vi "R30_1-RT.vi"() -> ()   [LabVIEW 2016]
uses:
  Controls/GP307 cluster.ctl
  Controls/Aperture states.ctl
  Controls/Faraday cup states.ctl
  Controls/Cryo Readback.ctl
  <vilib>/FPGAPlugInAG/cRIO-9067/niLvFpga_Open_cRIO-9067.vi
  <vilib>/rvi/interface/common/dynamic/niFpgaDynamicAddResources.vi
  <vilib>/Utility/error.llb/Error Cluster From Error Code.vi
  <vilib>/rvi/errors/niLvFpgaAdjustHostInterfaceError.vi
  <vilib>/rvi/interface/nirviOpenFPGA/nirviOpenFPGA.xnode
  PRIME Lab 2017a/Builds/cRIOs/R30-cRIO/FPGA/PRIMEControl2017_FPGA-R30_FPGA-R30_glZcTR5UBYc.lvbitx
  PRIME Lab 2017a/CONnie/PRIME Control 2017a/cRIO code/R30-1/R30_1-FPGA.vi
  <vilib>/rvi/interface/nirviReadWriteControl/nirviReadWriteControl.xnode
  <vilib>/NI_Real-Time Target Support.lvlib
  <vilib>/rvi/interface/Simulation/niFpgaSimulationCallBeginRW.vi
  NiFpgaLv.dll
panel:
  out "X+ Steerer V set":fxp<+/-,20,5>
  out "X- Steerer V set":fxp<+/-,20,5>
  out "Y+ Steerer V set":fxp<+/-,20,5>
  out "Y- Steerer V set":fxp<+/-,20,5>
  out "Cryo Readback":T1
  out "Time since re-purge":string
  out "2nd Stage Temp":string
  out "1st Stage Temp":string
  out "On-time":string
  out "Status":string
  in  "Tab Control":T2(tab)
  out "ESA I read":fxp<+/-,26,5>
  out "ESA V read":fxp<+/-,26,7>
  out "X- Steerer V read":fxp<+/-,26,7>
  out "Y+ Steerer I read":fxp<+/-,26,5>
  out "Y+ Steerer V read":fxp<+/-,26,7>
  out "Y- Steerer I read":fxp<+/-,26,5>
  out "Y- Steerer V read":fxp<+/-,26,7>
  out "X+ Steerer V read":fxp<+/-,26,7>
  out "X- Steerer I read":fxp<+/-,26,5>
  out "X+ Steerer I read":fxp<+/-,26,5>
  out "ESA Voltage set":fxp<+/-,20,5>
  out "Quad B I read":fxp<+/-,26,5>
  out "Quad A I read":fxp<+/-,26,5>
  out "Quad A set":fxp<+/-,20,5>
  out "Quad B set":fxp<+/-,20,5>
  out "Mag Steerer I-program":fxp<+/-,20,5>
  out "Mag Steerer V read":fxp<+/-,26,7>
  out "Mag Steerer I read":fxp<+/-,26,5>
  out "R30 Detector Ion gauge 1":u8[](array[numeric])
  out "R30 Detector Convectron  1":u8[](array[numeric])
  out "R30 ESA Ion gauge 1":u8[](array[numeric])
  out "Switch Image Convectron 1":u8[](array[numeric])
  out "Switch Image Ion Gauge 1":u8[](array[numeric])
  out "R30 ESA Convectron  1":u8[](array[numeric])
  out "Cryo 1st stage temp":u8[](array[numeric])
  out "Cryo On-time":u8[](array[numeric])
  out "Cryo status":u8[](array[numeric])
  out "Cryo 2nd stage temp":u8[](array[numeric])
  out "Time since repurge":u8[](array[numeric])
  out "ESA Vac cluster":T3
  out "Switch Image Vac Cluster":T3
  out "Detector Vac Cluster":T3
  out "Detector FC Status":T4
  out "Switch Image FC Status":T4
  out "Switch Image Aperture Status":T5
  out "Detector FC Position":cluster{"IN sensor":bool, "OUT sensor":bool}
  out "Detector Aperture Status":T5
  out "Switch Image FC Position":cluster{"IN sensor":bool, "OUT sensor":bool}
  out "Switch Image Aperture Position":cluster{"IN sensor":bool, "OUT sensor":bool}
  out "Detector Aperture Position":cluster{"IN sensor":bool, "OUT sensor":bool}
  out "Error Reporter":errorcluster
  out "HV control loop error":errorcluster
  out "HV readback loop error":errorcluster
  out "Actuator Sensor loop error":errorcluster
  out "Vac Cluster loop error":errorcluster
  out "Cryo loop error":errorcluster
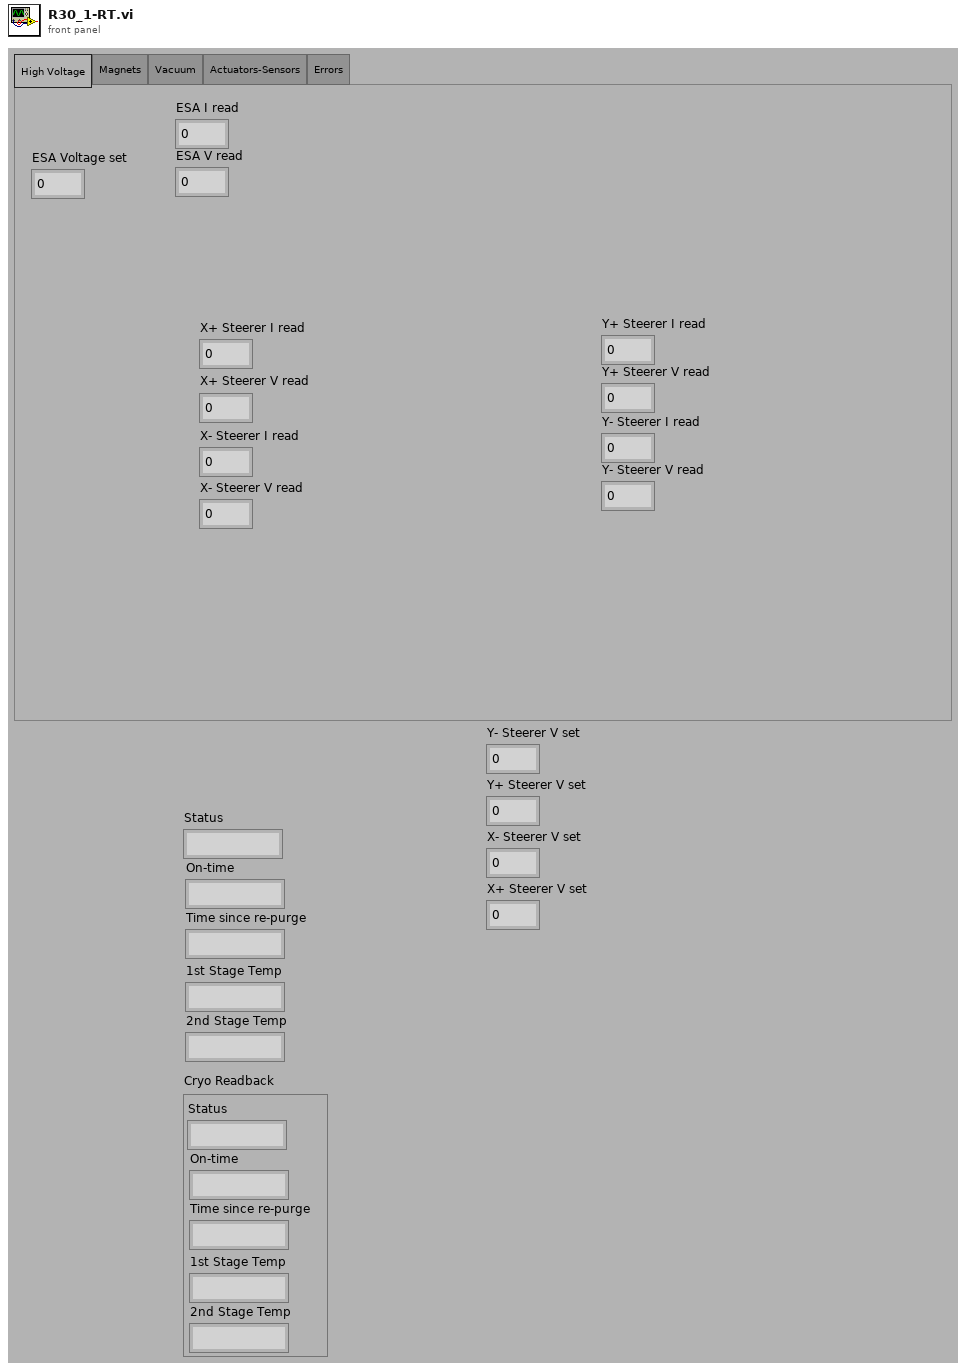
[diagram p1: front panel]
types:
  T1 = typedef "Cryo Readback.ctl" = cluster{"Status":string, "On-time":string, "1st Stage Temp":string, "2nd Stage Temp":string, "Time since re-purge":string}
  T2 = enum32{"High Voltage", "Magnets", "Vacuum", "Actuators-Sensors", "Errors"}
  T3 = typedef "GP307 cluster.ctl" = cluster{"Ion gauge 1":string, "Convectron  Gauge 1 ":string, "Ion Gauge 2":string, "Convectrom Gauge 2":string}
  T4 = typedef "Faraday cup states.ctl" = enum16{"FC status unclear", "FC in", "FC out"}
  T5 = typedef "Aperture states.ctl" = enum16{"Aperture status unclear", "Aperture in", "Aperture out"}
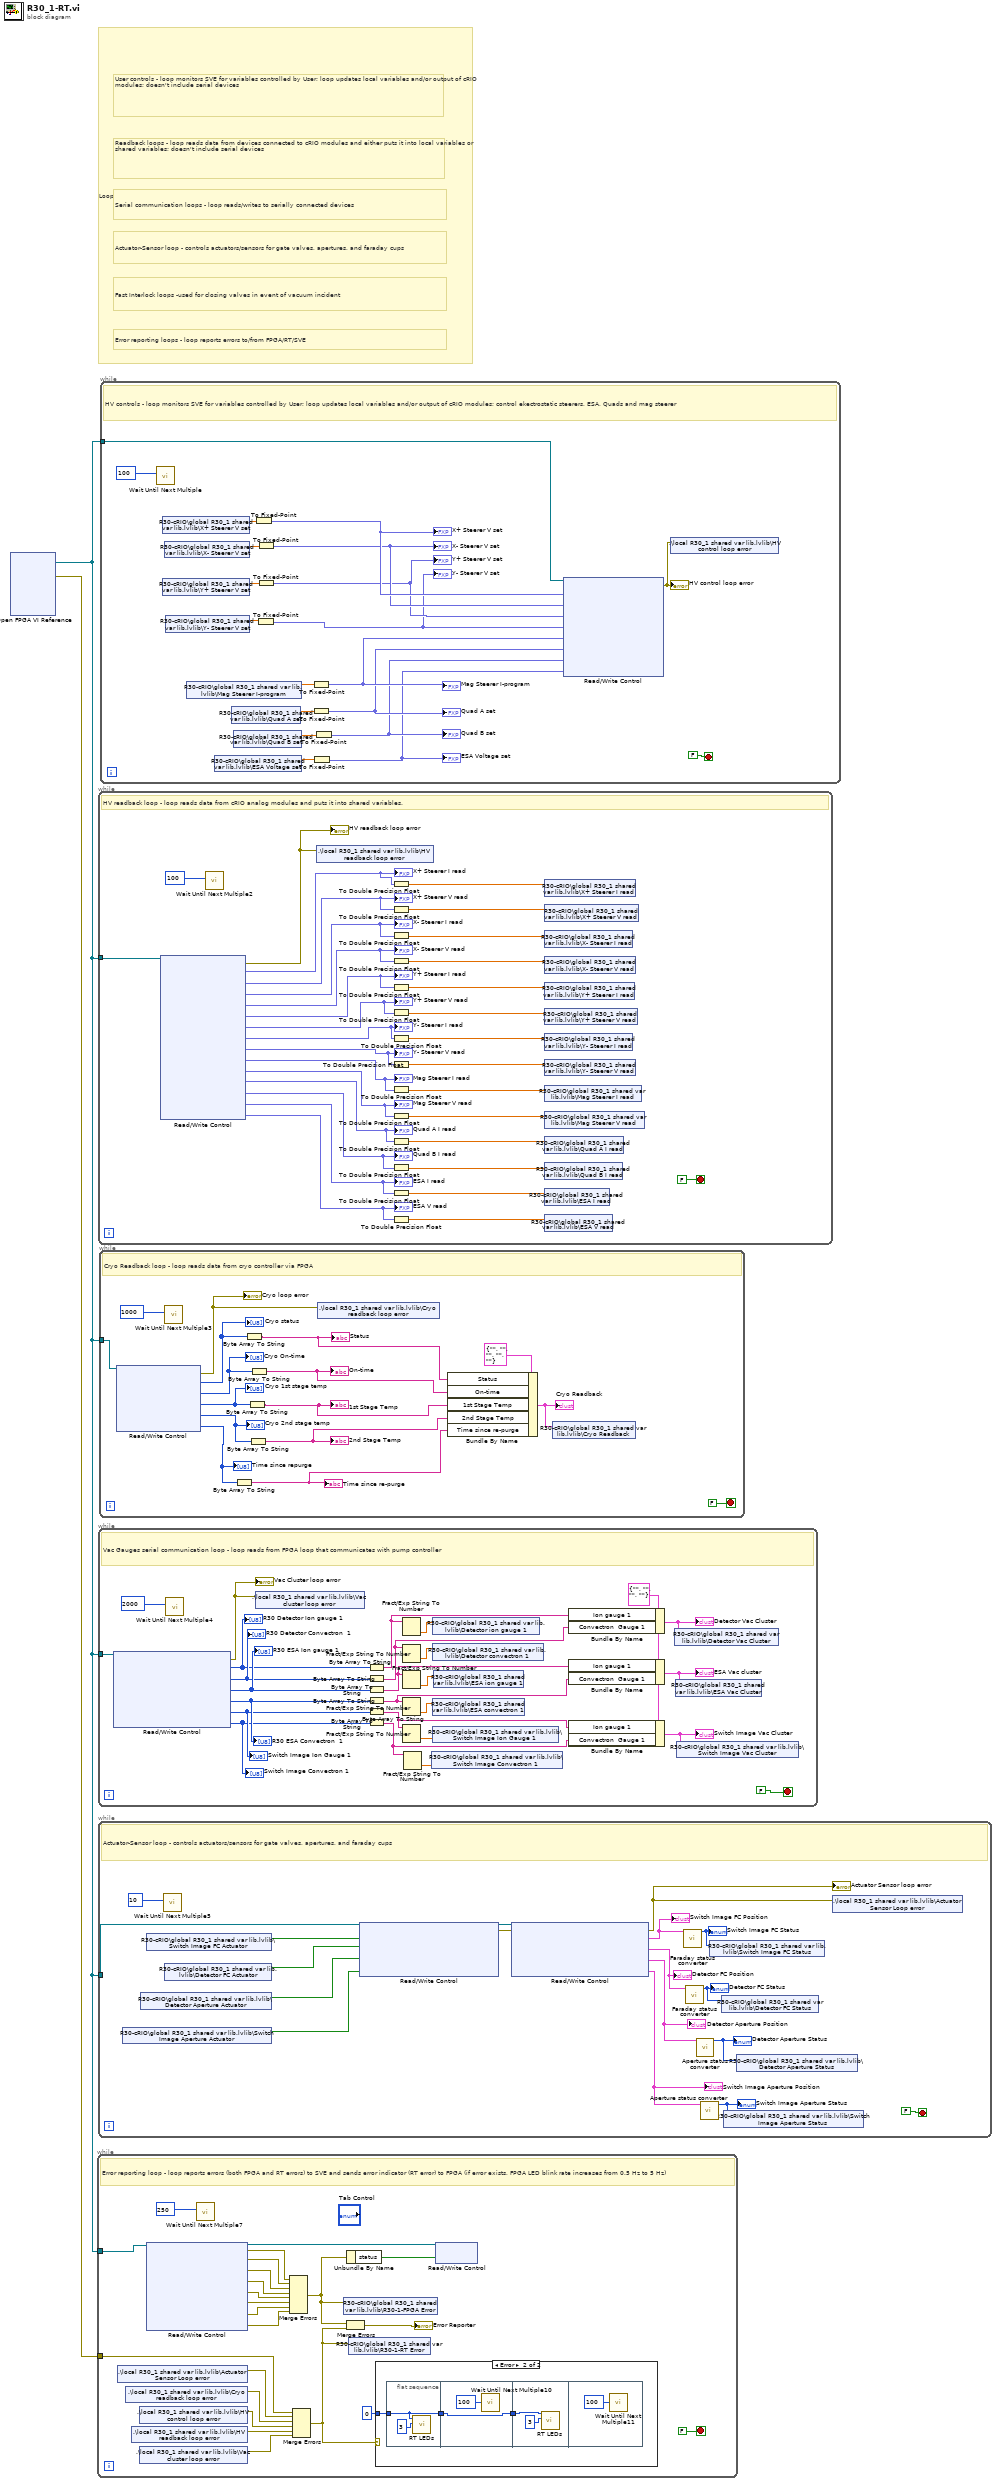
[diagram p0: block diagram]
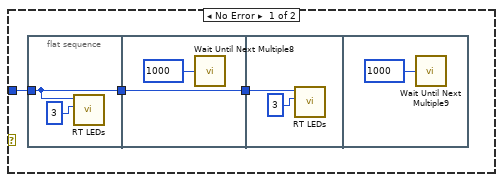
[diagram p2: hidden frame]
diagram:
  # "Actuator-Sensor loop - controls actuators/sensors for gate valves, apertures, and faraday cups"
  # "Fast Interlock loops -used for closing valves in event of vacuum incident"
  # "Error reporting loops - loop reports errors to/from FPGA/RT/SVE"
  # "Serial communication loops - loop reads/writes to serially connected devices"
  # "Readback loops - loop reads data from devices connected to cRIO modules and either puts it into local variables or shared variables; doesn't include serial devices"
  # "User controls - loop monitors SVE for variables controlled by User; loop updates local variables and/or output of cRIO modules; doesn't include serial devices"
  # "Loop legend - loops are color coded by responsibility"
  n1 = xnode "Open FPGA VI Reference"() -> ("FPGA VI Reference Out"=w1:refnum<k20>, "error out"=w2:errorcluster)  [unwired: 2 in]
  n2 = while {
    tunnel: w1 -> [w25]
    tunnel: w2 -> [w5]
    stop <- FALSE stop-if-true
    # "Error reporting loop - loop reports errors (both FPGA and RT errors) to SVE and sends error indicator (RT error) to FPGA (if error exists, FPGA LED blink rate increases from 0.5 Hz to 5 Hz)"
    n3 = shared-variable ".\\local R30_1 shared var lib.lvlib\\Actuator Sensor Loop error"() -> (w6:errorcluster)  [unwired: 1 in, 1 out]
    n4 = shared-variable ".\\local R30_1 shared var lib.lvlib\\Cryo readback loop error"() -> (w7:errorcluster)  [unwired: 1 in, 1 out]
    n5 = shared-variable ".\\local R30_1 shared var lib.lvlib\\HV readback loop error"() -> (w9:errorcluster)  [unwired: 1 in, 1 out]
    n6 = shared-variable ".\\local R30_1 shared var lib.lvlib\\HV control loop error"() -> (w8:errorcluster)  [unwired: 1 in, 1 out]
    n7 = shared-variable ".\\local R30_1 shared var lib.lvlib\\Vac cluster loop error"() -> (w10:errorcluster)  [unwired: 1 in, 1 out]
    n8 = xnode "Read/Write Control"("FPGA VI Reference In"=w25) -> ("FPGA VI Reference Out"=w17:refnum<k20>, "error out"=w24:errorcluster, "Vacuum Gauge 1 error"=w23:errorcluster, "Vacuum Gauge 2 error"=w22:errorcluster, "Vacuum Gauge 1 error"=w21:errorcluster, "Cryo Readback error"=w20:errorcluster, "HV control loop error"=w19:errorcluster, "Actuator loop error"=w18:errorcluster, "HV readback loop error"=w14:errorcluster)  [unwired: 1 in]
    n9 = call "Wait Until Next Multiple7"("Count(mSec)"=u32 250 ("millisecond multiple")) -> ()  [unwired: 1 out]
    n10 = Merge Errors(w24, w23, w22, w21, w20, w19, w18, w14) -> (w12:errorcluster)
    n11 = Merge Errors(w5, w6, w7, w8, w9, w10) -> (w3:errorcluster)
    n12 = shared-variable "R30-cRIO\\global R30_1 shared var lib.lvlib\\R30-1-FPGA Error"(w12) -> ()  [unwired: 1 in, 1 out]
    n13 = Unbundle By Name(w12) -> ("status"=w16:bool)
    n14 = Merge Errors(w12, w3) -> (→"Error Reporter":errorcluster)
    n15 = shared-variable "R30-cRIO\\global R30_1 shared var lib.lvlib\\R30-1-RT Error"(w3) -> ()  [unwired: 1 in, 1 out]
    n16 = case shown="Error" w3 {
      tunnel: 0 -> [w28 w36]
      frame No Error {
        n17 = flat-sequence {
          tunnel: w28 -> [w29]
          tunnel: [w29] -> w26
          tunnel: [w31] -> w27
          tunnel: w26 -> [w31]
          tunnel: w27 -> [w33]
          frame #0 {
            n18 = call <vilib>:"RT LEDs.vi"("State"=3, "LED Num"=w29) -> ()  [unwired: 4 in, 2 out]
          }
          frame #1 {
            n19 = call "Wait Until Next Multiple8"("Count(mSec)"=u16 1000) -> ()  [unwired: 1 out]
          }
          frame #2 {
            n20 = call <vilib>:"RT LEDs.vi"("State"=3, "LED Num"=w33) -> ()  [unwired: 4 in, 2 out]
          }
          frame #3 {
            n21 = call "Wait Until Next Multiple9"("Count(mSec)"=u16 1000) -> ()  [unwired: 1 out]
          }
        }
      }
      frame Error {
        n22 = flat-sequence {
          tunnel: [w39] -> w38
          tunnel: w36 -> [w39]
          tunnel: w38 -> [w41]
          tunnel: [w41] -> w37
          tunnel: w37 -> [w43]
          frame #0 {
            n23 = call <vilib>:"RT LEDs.vi"("State"=3, "LED Num"=w39) -> ()  [unwired: 4 in, 2 out]
          }
          frame #1 {
            n24 = call "Wait Until Next Multiple10"("Count(mSec)"=u16 100) -> ()  [unwired: 1 out]
          }
          frame #2 {
            n25 = call <vilib>:"RT LEDs.vi"("State"=3, "LED Num"=w43) -> ()  [unwired: 4 in, 2 out]
          }
          frame #3 {
            n26 = call "Wait Until Next Multiple11"("Count(mSec)"=u16 100) -> ()  [unwired: 1 out]
          }
        }
      }
    }
    n27 = xnode "Read/Write Control"("FPGA VI Reference In"=w17, "RT error"=w16) -> ()  [unwired: 1 in, 2 out]
  }
  n28 = while {
    tunnel: w1 -> [w76]
    stop <- FALSE stop-if-true
    # "HV readback loop - loop reads data from cRIO analog modules and puts it into shared variables."
    n29 = xnode "Read/Write Control"("FPGA VI Reference In"=w76) -> ("error out"=w75:errorcluster, "X+ Steerer I read"=w74:fxp<+/-,26,5>, "X+ Steerer V read"=w73:fxp<+/-,26,5>, "X- Steerer I read"=w72:fxp<+/-,26,5>, "X- Steerer V read"=w71:fxp<+/-,26,5>, "Y+ Steerer I read"=w70:fxp<+/-,26,5>, "Y+ Steerer V read"=w69:fxp<+/-,26,5>, "Y- Steerer I read"=w68:fxp<+/-,26,5>, "Y- Steerer V read"=w67:fxp<+/-,26,5>, "Mag Steerer I read"=w66:fxp<+/-,26,5>, "Mag Steerer V read"=w65:fxp<+/-,26,5>, "Quad A I read"=w64:fxp<+/-,26,5>, "Quad B I read"=w63:fxp<+/-,26,5>, "ESA I read"=w62:fxp<+/-,26,5>, "ESA V read"=w61:fxp<+/-,26,5>)  [unwired: 1 in, 1 out]
    "HV readback loop error" <- w75
    "X+ Steerer I read" <- w74
    "X+ Steerer V read" <- w73
    "X- Steerer I read" <- w72
    "X- Steerer V read" <- w71
    "Y+ Steerer I read" <- w70
    "Y+ Steerer V read" <- w69
    "Y- Steerer I read" <- w68
    "Y- Steerer V read" <- w67
    "Mag Steerer I read" <- w66
    "Mag Steerer V read" <- w65
    "Quad A I read" <- w64
    "Quad B I read" <- w63
    "ESA I read" <- w62
    "ESA V read" <- w61
    n30 = call "Wait Until Next Multiple2"("Count(mSec)"=u32 100 ("millisecond multiple")) -> ()  [unwired: 1 out]
    n31 = shared-variable ".\\local R30_1 shared var lib.lvlib\\HV readback loop error"(w75) -> ()  [unwired: 1 in, 1 out]
    n32 = To Double Precision Float(number=w74) -> (double precision float=w47:dbl)
    n33 = To Double Precision Float(number=w73) -> (double precision float=w48:dbl)
    n34 = To Double Precision Float(number=w72) -> (double precision float=w49:dbl)
    n35 = To Double Precision Float(number=w71) -> (double precision float=w50:dbl)
    n36 = To Double Precision Float(number=w70) -> (double precision float=w51:dbl)
    n37 = To Double Precision Float(number=w69) -> (double precision float=w52:dbl)
    n38 = To Double Precision Float(number=w68) -> (double precision float=w53:dbl)
    n39 = To Double Precision Float(number=w67) -> (double precision float=w54:dbl)
    n40 = To Double Precision Float(number=w66) -> (double precision float=w60:dbl)
    n41 = To Double Precision Float(number=w65) -> (double precision float=w59:dbl)
    n42 = To Double Precision Float(number=w64) -> (double precision float=w58:dbl)
    n43 = To Double Precision Float(number=w63) -> (double precision float=w57:dbl)
    n44 = To Double Precision Float(number=w62) -> (double precision float=w56:dbl)
    n45 = To Double Precision Float(number=w61) -> (double precision float=w55:dbl)
    n46 = shared-variable "R30-cRIO\\global R30_1 shared var lib.lvlib\\X+ Steerer I read"(w47) -> ()  [unwired: 1 in, 1 out]
    n47 = shared-variable "R30-cRIO\\global R30_1 shared var lib.lvlib\\X+ Steerer V read"(w48) -> ()  [unwired: 1 in, 1 out]
    n48 = shared-variable "R30-cRIO\\global R30_1 shared var lib.lvlib\\X- Steerer I read"(w49) -> ()  [unwired: 1 in, 1 out]
    n49 = shared-variable "R30-cRIO\\global R30_1 shared var lib.lvlib\\X- Steerer V read"(w50) -> ()  [unwired: 1 in, 1 out]
    n50 = shared-variable "R30-cRIO\\global R30_1 shared var lib.lvlib\\Y+ Steerer I read"(w51) -> ()  [unwired: 1 in, 1 out]
    n51 = shared-variable "R30-cRIO\\global R30_1 shared var lib.lvlib\\Y+ Steerer V read"(w52) -> ()  [unwired: 1 in, 1 out]
    n52 = shared-variable "R30-cRIO\\global R30_1 shared var lib.lvlib\\Y- Steerer I read"(w53) -> ()  [unwired: 1 in, 1 out]
    n53 = shared-variable "R30-cRIO\\global R30_1 shared var lib.lvlib\\Y- Steerer V read"(w54) -> ()  [unwired: 1 in, 1 out]
    n54 = shared-variable "R30-cRIO\\global R30_1 shared var lib.lvlib\\Mag Steerer I read"(w60) -> ()  [unwired: 1 in, 1 out]
    n55 = shared-variable "R30-cRIO\\global R30_1 shared var lib.lvlib\\Mag Steerer V read"(w59) -> ()  [unwired: 1 in, 1 out]
    n56 = shared-variable "R30-cRIO\\global R30_1 shared var lib.lvlib\\Quad A I read"(w58) -> ()  [unwired: 1 in, 1 out]
    n57 = shared-variable "R30-cRIO\\global R30_1 shared var lib.lvlib\\Quad B I read"(w57) -> ()  [unwired: 1 in, 1 out]
    n58 = shared-variable "R30-cRIO\\global R30_1 shared var lib.lvlib\\ESA I read"(w56) -> ()  [unwired: 1 in, 1 out]
    n59 = shared-variable "R30-cRIO\\global R30_1 shared var lib.lvlib\\ESA V read"(w55) -> ()  [unwired: 1 in, 1 out]
  }
  n60 = while {
    tunnel: w1 -> [w103]
    stop <- FALSE stop-if-true
    w93 = T3 {"Ion gauge 1"="", "Convectron  Gauge 1 "="", "Ion Gauge 2"="", "Convectrom Gauge 2"=""} ("Ion gauge cluster control")
    # "Vac Gauges serial communication loop - loop reads from FPGA loop that communicates with pump controller"
    n61 = xnode "Read/Write Control"("FPGA VI Reference In"=w103) -> ("error out"=w79:errorcluster, "R30 Detector Ion gauge 1"=w98:u8[], "R30 Detector Convectron  1"=w99:u8[], "R30 ESA Ion gauge 1"=w100:u8[], "R30 ESA Convectron  1"=w101:u8[], "Switch Image Ion Gauge 1"=w92:u8[], "Switch Image Convectron 1"=w91:u8[])  [unwired: 1 in, 1 out]
    "R30 Detector Ion gauge 1" <- w98
    "R30 Detector Convectron  1" <- w99
    "R30 ESA Ion gauge 1" <- w100
    "Switch Image Convectron 1" <- w91
    "Switch Image Ion Gauge 1" <- w92
    "R30 ESA Convectron  1" <- w101
    "Vac Cluster loop error" <- w79
    n62 = call "Wait Until Next Multiple4"("Count(mSec)"=u32 2000 ("millisecond multiple")) -> ()  [unwired: 1 out]
    n63 = shared-variable ".\\local R30_1 shared var lib.lvlib\\Vac cluster loop error"(w79) -> ()  [unwired: 1 in, 1 out]
    n64 = Byte Array To String(unsigned byte array=w98) -> (string=w90:string)
    n65 = Byte Array To String(unsigned byte array=w99) -> (string=w89:string)
    n66 = Byte Array To String(unsigned byte array=w100) -> (string=w88:string)
    n67 = Byte Array To String(unsigned byte array=w101) -> (string=w87:string)
    n68 = Byte Array To String(unsigned byte array=w92) -> (string=w84:string)
    n69 = Byte Array To String(unsigned byte array=w91) -> (string=w83:string)
    n70 = Fract/Exp String To Number(string=w90) -> (number=w95:dbl)  [unwired: 3 in, 1 out]
    n71 = Fract/Exp String To Number(string=w89) -> (number=w94:dbl)  [unwired: 3 in, 1 out]
    n72 = Fract/Exp String To Number(string=w88) -> (number=w97:dbl)  [unwired: 3 in, 1 out]
    n73 = Fract/Exp String To Number(string=w87) -> (number=w96:dbl)  [unwired: 3 in, 1 out]
    n74 = Fract/Exp String To Number(string=w84) -> (number=w86:dbl)  [unwired: 3 in, 1 out]
    n75 = Fract/Exp String To Number(string=w83) -> (number=w85:dbl)  [unwired: 3 in, 1 out]
    n76 = shared-variable "R30-cRIO\\global R30_1 shared var lib.lvlib\\Switch Image Convectron 1"(w85) -> ()  [unwired: 1 in, 1 out]
    n77 = shared-variable "R30-cRIO\\global R30_1 shared var lib.lvlib\\Detector ion gauge 1"(w95) -> ()  [unwired: 1 in, 1 out]
    n78 = shared-variable "R30-cRIO\\global R30_1 shared var lib.lvlib\\Detector convectron 1"(w94) -> ()  [unwired: 1 in, 1 out]
    n79 = shared-variable "R30-cRIO\\global R30_1 shared var lib.lvlib\\ESA convectron 1"(w96) -> ()  [unwired: 1 in, 1 out]
    n80 = shared-variable "R30-cRIO\\global R30_1 shared var lib.lvlib\\Switch Image Ion Gauge 1"(w86) -> ()  [unwired: 1 in, 1 out]
    n81 = shared-variable "R30-cRIO\\global R30_1 shared var lib.lvlib\\ESA ion gauge 1"(w97) -> ()  [unwired: 1 in, 1 out]
    n82 = Bundle By Name(cluster=w93, "Ion gauge 1"=w90, "Convectron  Gauge 1"=w89) -> (w80:T3)
    "Detector Vac Cluster" <- w80
    n83 = Bundle By Name(cluster=w93, "Ion gauge 1"=w88, "Convectron  Gauge 1"=w87) -> (w81:T3)
    "ESA Vac cluster" <- w81
    n84 = Bundle By Name(cluster=w93, "Ion gauge 1"=w84, "Convectron  Gauge 1"=w83) -> (w82:T3)
    "Switch Image Vac Cluster" <- w82
    n85 = shared-variable "R30-cRIO\\global R30_1 shared var lib.lvlib\\Detector Vac Cluster"(w80) -> ()  [unwired: 1 in, 1 out]
    n86 = shared-variable "R30-cRIO\\global R30_1 shared var lib.lvlib\\ESA Vac Cluster"(w81) -> ()  [unwired: 1 in, 1 out]
    n87 = shared-variable "R30-cRIO\\global R30_1 shared var lib.lvlib\\Switch Image Vac Cluster"(w82) -> ()  [unwired: 1 in, 1 out]
  }
  n88 = while {
    tunnel: w1 -> [w105]
    stop <- FALSE stop-if-true
    # "Actuator-Sensor loop - controls actuators/sensors for gate valves, apertures, and faraday cups"
    n89 = shared-variable "R30-cRIO\\global R30_1 shared var lib.lvlib\\Switch Image Aperture Actuator"() -> (w114:bool)  [unwired: 1 in, 1 out]
    n90 = shared-variable "R30-cRIO\\global R30_1 shared var lib.lvlib\\Detector Aperture Actuator"() -> (w115:bool)  [unwired: 1 in, 1 out]
    n91 = shared-variable "R30-cRIO\\global R30_1 shared var lib.lvlib\\Switch Image FC Actuator"() -> (w117:bool)  [unwired: 1 in, 1 out]
    n92 = call "Wait Until Next Multiple5"("Count(mSec)"=u32 10 ("millisecond multiple")) -> ()  [unwired: 1 out]
    n93 = shared-variable "R30-cRIO\\global R30_1 shared var lib.lvlib\\Detector FC Actuator"() -> (w116:bool)  [unwired: 1 in, 1 out]
    n94 = xnode "Read/Write Control"("FPGA VI Reference In"=w105, "Switch magnet FC Actuator"=w117, "Detector FC Actuator"=w116, "Detector Aperture Actuator"=w115, "Switch magnet Aperture Actuator"=w114) -> ("FPGA VI Reference Out"=w120:refnum<k20>, "error out"=w119:errorcluster)  [unwired: 1 in]
    n95 = xnode "Read/Write Control"("FPGA VI Reference In"=w120, "error in"=w119) -> ("error out"=w118:errorcluster, "Switch Magnet FC Position"=w107:cluster{"IN sensor":bool, "OUT sensor":bool}, "Detector FC Position"=w109:cluster{"IN sensor":bool, "OUT sensor":bool}, "Detector Aperture Position"=w108:cluster{"IN sensor":bool, "OUT sensor":bool}, "Switch Magnet Aperture Position"=w111:cluster{"IN sensor":bool, "OUT sensor":bool})  [unwired: 1 out]
    "Actuator Sensor loop error" <- w118
    "Switch Image FC Position" <- w107
    "Switch Image Aperture Position" <- w111
    "Detector Aperture Position" <- w108
    "Detector FC Position" <- w109
    n96 = call "Faraday status converter.vi"("FC Position"=w107) -> ("FC Status"=w112:T4)  [unwired: 10 in]
    "Switch Image FC Status" <- w112
    n97 = call "Faraday status converter.vi"("FC Position"=w109) -> ("FC Status"=w106:T4)  [unwired: 10 in]
    "Detector FC Status" <- w106
    n98 = call "Aperture status converter.vi"("Aperture Position"=w108) -> ("Aperture Status"=w110:T5)  [unwired: 10 in]
    "Detector Aperture Status" <- w110
    n99 = call "Aperture status converter.vi"("Aperture Position"=w111) -> ("Aperture Status"=w113:T5)  [unwired: 10 in]
    "Switch Image Aperture Status" <- w113
    n100 = shared-variable "R30-cRIO\\global R30_1 shared var lib.lvlib\\Switch Image FC Status"(w112) -> ()  [unwired: 1 in, 1 out]
    n101 = shared-variable "R30-cRIO\\global R30_1 shared var lib.lvlib\\Detector FC Status"(w106) -> ()  [unwired: 1 in, 1 out]
    n102 = shared-variable "R30-cRIO\\global R30_1 shared var lib.lvlib\\Switch Image Aperture Status"(w113) -> ()  [unwired: 1 in, 1 out]
    n103 = shared-variable "R30-cRIO\\global R30_1 shared var lib.lvlib\\Detector Aperture Status"(w110) -> ()  [unwired: 1 in, 1 out]
    n104 = shared-variable ".\\local R30_1 shared var lib.lvlib\\Actuator Sensor Loop error"(w118) -> ()  [unwired: 1 in, 1 out]
  }
  n105 = while {
    tunnel: w1 -> [w136]
    stop <- FALSE stop-if-true
    # "Cryo Readback loop - loop reads data from cryo controller via FPGA"
    n106 = xnode "Read/Write Control"("FPGA VI Reference In"=w136) -> ("error out"=w130:errorcluster, "Cryo Status"=w133:u8[], "Cryo On-time"=w134:u8[], "1st stage temp"=w135:u8[], "2nd stage temp"=w132:u8[], "Time since repurge"=w131:u8[])  [unwired: 1 in, 1 out]
    "Cryo status" <- w133
    "Cryo On-time" <- w134
    "Cryo 1st stage temp" <- w135
    "Cryo loop error" <- w130
    "Cryo 2nd stage temp" <- w132
    "Time since repurge" <- w131
    n107 = call "Wait Until Next Multiple3"("Count(mSec)"=u32 1000 ("millisecond multiple")) -> ()  [unwired: 1 out]
    n108 = Byte Array To String(unsigned byte array=w131) -> (string=w122:string)
    "Time since re-purge" <- w122
    n109 = Byte Array To String(unsigned byte array=w133) -> (string=w126:string)
    "Status" <- w126
    n110 = Byte Array To String(unsigned byte array=w135) -> (string=w124:string)
    "1st Stage Temp" <- w124
    n111 = Byte Array To String(unsigned byte array=w132) -> (string=w123:string)
    "2nd Stage Temp" <- w123
    n112 = Byte Array To String(unsigned byte array=w134) -> (string=w125:string)
    "On-time" <- w125
    n113 = shared-variable ".\\local R30_1 shared var lib.lvlib\\Cryo readback loop error"(w130) -> ()  [unwired: 1 in, 1 out]
    n114 = Bundle By Name(cluster=T1 {"Status"="", "On-time"="", "1st Stage Temp"="", "2nd Stage Temp"="", "Time since re-purge"=""} ("Cryo Readback"), "Status"=w126, "On-time"=w125, "1st Stage Temp"=w124, "2nd Stage Temp"=w123, "Time since re-purge"=w122) -> (w127:T1)
    "Cryo Readback" <- w127
    n115 = shared-variable "R30-cRIO\\global R30_1 shared var lib.lvlib\\Cryo Readback"(w127) -> ()  [unwired: 1 in, 1 out]
  }
  n116 = while {
    tunnel: w1 -> [w148]
    stop <- FALSE stop-if-true
    # "HV controls - loop monitors SVE for variables controlled by User; loop updates local variables and/or output of cRIO modules; control ekectrostatic steerers, ESA, Quads and mag steerer"
    n117 = call "Wait Until Next Multiple"("Count(mSec)"=u32 100 ("millisecond multiple")) -> ()  [unwired: 1 out]
    n118 = shared-variable "R30-cRIO\\global R30_1 shared var lib.lvlib\\X+ Steerer V set"() -> (w144:dbl)  [unwired: 1 in, 1 out]
    n119 = shared-variable "R30-cRIO\\global R30_1 shared var lib.lvlib\\Y+ Steerer V set"() -> (w146:dbl)  [unwired: 1 in, 1 out]
    n120 = shared-variable "R30-cRIO\\global R30_1 shared var lib.lvlib\\X- Steerer V set"() -> (w145:dbl)  [unwired: 1 in, 1 out]
    n121 = shared-variable "R30-cRIO\\global R30_1 shared var lib.lvlib\\Y- Steerer V set"() -> (w147:dbl)  [unwired: 1 in, 1 out]
    n122 = shared-variable "R30-cRIO\\global R30_1 shared var lib.lvlib\\Mag Steerer I-program"() -> (w156:dbl)  [unwired: 1 in, 1 out]
    n123 = shared-variable "R30-cRIO\\global R30_1 shared var lib.lvlib\\ESA Voltage set"() -> (w150:dbl)  [unwired: 1 in, 1 out]
    n124 = shared-variable "R30-cRIO\\global R30_1 shared var lib.lvlib\\Quad A set"() -> (w154:dbl)  [unwired: 1 in, 1 out]
    n125 = shared-variable "R30-cRIO\\global R30_1 shared var lib.lvlib\\Quad B set"() -> (w152:dbl)  [unwired: 1 in, 1 out]
    n126 = To Fixed-Point(number=w144) -> (fixed-point=w141:fxp<+/-,20,5>)  [unwired: 1 in]
    "X+ Steerer V set" <- w141
    n127 = To Fixed-Point(number=w147) -> (fixed-point=w138:fxp<+/-,20,5>)  [unwired: 1 in]
    "Y- Steerer V set" <- w138
    n128 = To Fixed-Point(number=w145) -> (fixed-point=w140:fxp<+/-,20,5>)  [unwired: 1 in]
    "X- Steerer V set" <- w140
    n129 = To Fixed-Point(number=w146) -> (fixed-point=w139:fxp<+/-,20,5>)  [unwired: 1 in]
    "Y+ Steerer V set" <- w139
    n130 = To Fixed-Point(number=w156) -> (fixed-point=w155:fxp<+/-,20,5>)  [unwired: 1 in]
    "Mag Steerer I-program" <- w155
    n131 = To Fixed-Point(number=w154) -> (fixed-point=w153:fxp<+/-,20,5>)  [unwired: 1 in]
    "Quad A set" <- w153
    n132 = To Fixed-Point(number=w150) -> (fixed-point=w149:fxp<+/-,20,5>)  [unwired: 1 in]
    "ESA Voltage set" <- w149
    n133 = To Fixed-Point(number=w152) -> (fixed-point=w151:fxp<+/-,20,5>)  [unwired: 1 in]
    "Quad B set" <- w151
    n134 = xnode "Read/Write Control"("FPGA VI Reference In"=w148, "X+ Steerer V set"=w141, "X- Steerer V set"=w140, "Y+ Steerer V set"=w139, "Y- Steerer V set"=w138, "Mag Steerer I-program"=w155, "Quad A set"=w153, "Quad B set"=w151, "ESA Voltage set"=w149) -> ("error out"=w143:errorcluster)  [unwired: 1 in, 1 out]
    "HV control loop error" <- w143
    n135 = shared-variable ".\\local R30_1 shared var lib.lvlib\\HV control loop error"(w143) -> ()  [unwired: 1 in, 1 out]
  }
